vi "getB2.vi"(3 "error in (no error)":errorcluster) -> (0 "error out":errorcluster, 2 "B-Feld":dbl)   [LabVIEW 2009]
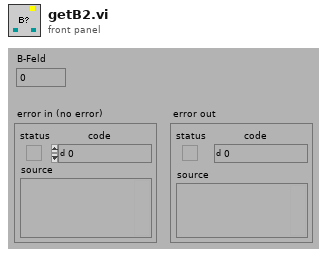
[diagram p1: front panel]
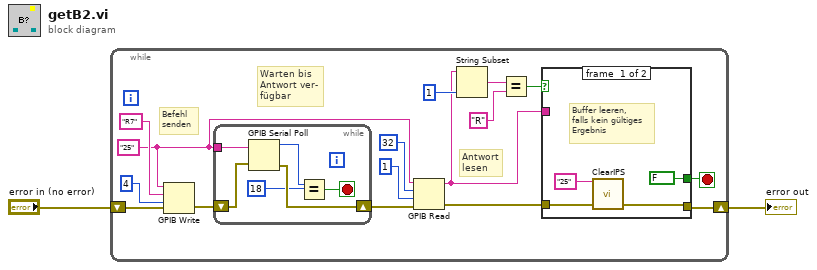
[diagram p0: block diagram]
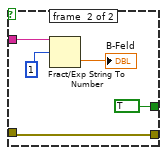
[diagram p2: hidden frame]
diagram:
  n1 = while {
    shift-right: [w3] -> w1
    shift-left: "error in (no error)" -> [w16]
    stop <- w5 stop-if-true
    w11 = "25"
    # "Antwort\nlesen"
    # "Warten bis\nAntwort ver-\nfügbar"
    # "Befehl\nsenden"
    n2 = GPIB Write(0:w11, 1:"R7", 2:4, 3:w16) -> (6:w15:errorcluster)  [unwired: 1 in, 1 out]
    n3 = while {
      shift-right: [w32] -> w14
      shift-left: w15 -> [w33]
      tunnel: w11 -> [w31]
      stop <- w30 stop-if-true
      n4 = GPIB Serial Poll(0:w31, 1:w33) -> (2:w28:i16, 4:w32:errorcluster)  [unwired: 1 out]
      n5 = Equal?(x=w28, y=18) -> (x = y?=w30:bool)
    }
    n6 = GPIB Read(0:w11, 1:32, 2:1, 3:w14) -> (5:w6:string, 7:w4:errorcluster)  [unwired: 1 in, 1 out]
    n7 = String Subset(string=w6, length (rest)=1) -> (substring=w9:string)  [unwired: 1 in]
    n8 = Equal?(x=w9, y="R") -> (x = y?=w7:bool)
    n9 = case shown="True" w7 {
      tunnel: w6 -> [_ w26]
      tunnel: [FALSE TRUE] -> w5
      tunnel: [w19 w23] -> w3
      tunnel: w4 -> [w20 w23]
      frame #0 {
        # "Buffer leeren,\nfalls kein gültiges\nErgebnis"
        n10 = call "ClearIPS.vi"("error in (no error)"=w20, "address string (25)"="25") -> ("error out"=w19:errorcluster)  [unwired: 3 in]
      }
      frame #1 {
        n11 = Fract/Exp String To Number(string=w26, offset=1) -> (number=→"B-Feld":dbl)  [unwired: 2 in, 1 out]
      }
    }
  }
  "error out" <- w1
